vi "IdleState.vi"(8 "error in (no error)":errorcluster, 9 "Cluster in":T2, 10 "Enum in":T1, 11 "Actual Start [i]":i64) -> (0 "error out":errorcluster, 2 "Cluster out":T2, 3 "Enum":T1)   [LabVIEW 2018]
uses:
  Type_Def/Type_Def Actuator Controls.ctl
  Type_Def/Type_Def ControlState.ctl
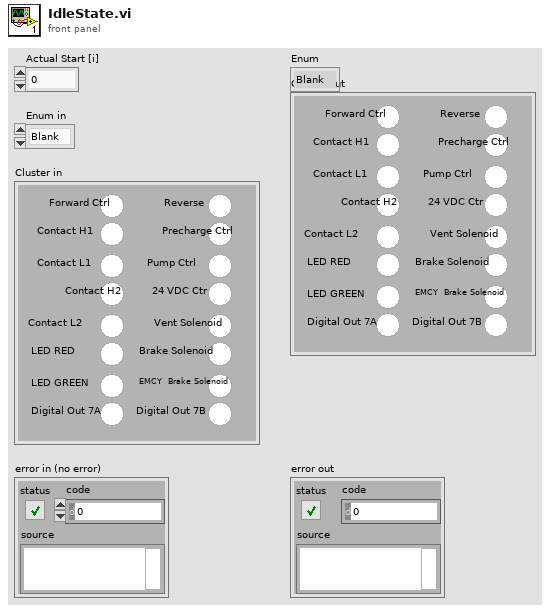
[diagram p1: front panel]
types:
  T1 = typedef "Type_Def ControlState.ctl" = enum16{"Blank", "Systems Check", "Idle", "Ready", "Pushing", "CrawlingPrecharge", "Braking", "Fault", "Boot Up", "Unpowered", "Crawling", "Shutdown", "Service Push", "Service Wait", "Vent", "Precharge", "Cooldown"}
  T2 = typedef "Type_Def Actuator Controls.ctl" = cluster{"Reverse ":bool, "Precharge Ctrl":bool, "Pump Ctrl":bool, "24 VDC Ctr":bool, "Vent Solenoid":bool, "Brake Solenoid":bool, "EMCY  Brake Solenoid":bool, "Digital Out 7B ":bool, "Forward Ctrl":bool, "Contact H1":bool, "Contact L1":bool, "Contact H2":bool, "Contact L2 ":bool, "LED RED":bool, "LED GREEN":bool, " Digital Out 7A":bool}
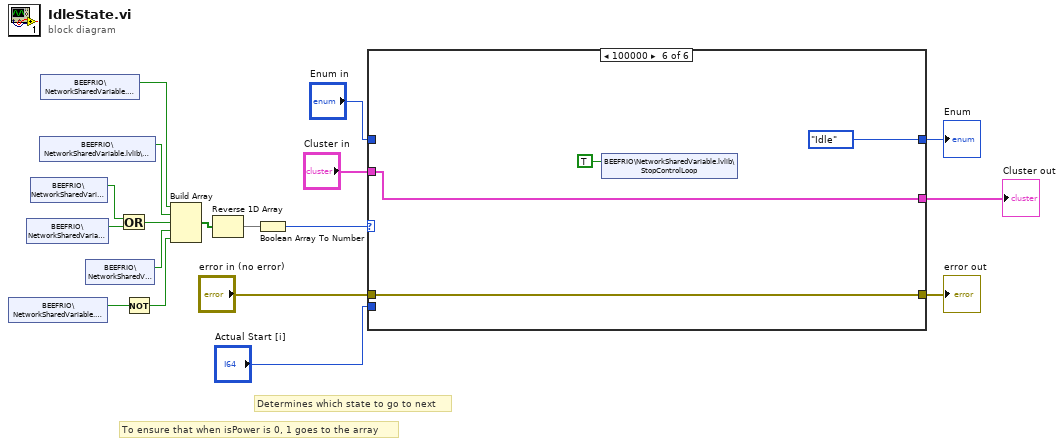
[diagram p0: block diagram]
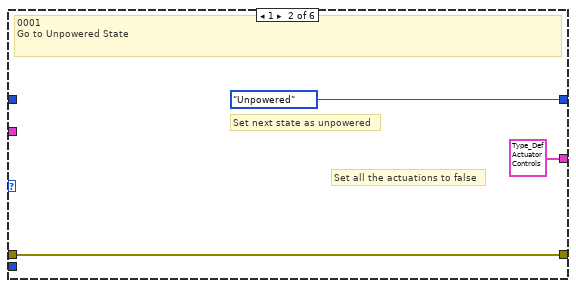
[diagram p3: hidden frame]
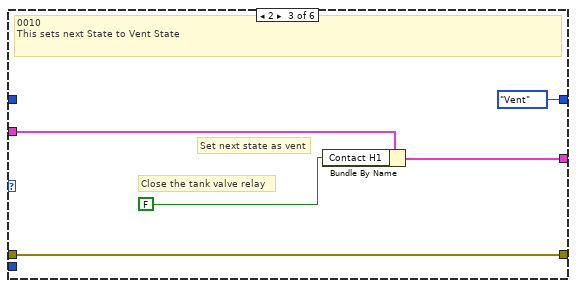
[diagram p4: hidden frame]
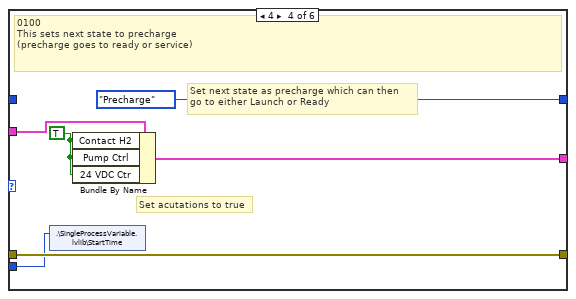
[diagram p5: hidden frame]
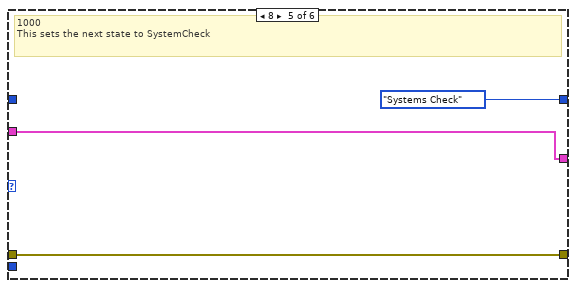
[diagram p6: hidden frame]
diagram:
  # "To ensure that when isPower is 0, 1 goes to the array"
  # "Determines which state to go to next"
  n1 = shared-variable "BEEFRIO\\NetworkSharedVariable.lvlib\\IsPowered"() -> (w11:bool)  [unwired: 1 in, 1 out]
  n2 = shared-variable "BEEFRIO\\NetworkSharedVariable.lvlib\\Service"() -> (w13:bool)  [unwired: 1 in, 1 out]
  n3 = shared-variable "BEEFRIO\\NetworkSharedVariable.lvlib\\Ready"() -> (w14:bool)  [unwired: 1 in, 1 out]
  n4 = shared-variable "BEEFRIO\\NetworkSharedVariable.lvlib\\SystemCheck"() -> (w2:bool)  [unwired: 1 in, 1 out]
  n5 = shared-variable "BEEFRIO\\NetworkSharedVariable.lvlib\\Shutdown"() -> (w1:bool)  [unwired: 1 in, 1 out]
  n6 = shared-variable "BEEFRIO\\NetworkSharedVariable.lvlib\\Vent"() -> (w7:bool)  [unwired: 1 in, 1 out]
  n7 = Or(x=w14, y=w13) -> (x .or. y?=w15:bool)
  n8 = Not(x=w11) -> (.not. x?=w12:bool)
  n9 = Build Array(w1, w2, w15, w7, w12) -> (w8:bool[])
  n10 = Reverse 1D Array(array=w8) -> (reversed array=w9:bool[])
  n11 = Boolean Array To Number(Boolean array=w9) -> (number=w10:u32)
  n12 = case shown="100000" w10 {
    tunnel: "Enum in" -> [w21 _ _ _ _ _]
    tunnel: [w21 Type_Def_ControlState."Unpowered" Type_Def_ControlState."Vent" Type_Def_ControlState."Precharge" Type_Def_ControlState."Systems Check" Type_Def_ControlState."Idle" ("Enum in")] -> w4
    tunnel: "Cluster in" -> [w20 _ w26 w34 w37 w42]
    tunnel: [w20 T2 {"Reverse "=FALSE, "Precharge Ctrl"=FALSE, "Pump Ctrl"=FALSE, "24 VDC Ctr"=FALSE, "Vent Solenoid"=FALSE, "Brake Solenoid"=FALSE, "EMCY  Brake Solenoid"=FALSE, "Digital Out 7B "=FALSE, "Forward Ctrl"=FALSE, "Contact H1"=FALSE, "Contact L1"=FALSE, "Contact H2"=FALSE, "Contact L2 "=FALSE, "LED RED"=FALSE, "LED GREEN"=FALSE, " Digital Out 7A"=FALSE} w27 w32 w37 w42] -> w6
    tunnel: [w19 w22 w25 w31 w36 w40] -> w16
    tunnel: "error in (no error)" -> [w19 w22 w25 w31 w36 w40]
    tunnel: "Actual Start [i]" -> [_ _ _ w30 _ _]
    frame 0, Default {
      # "Does nothing and stays in Idle mode"
    }
    frame 1 {
      # "Set next state as unpowered"
      # "Set all the actuations to false"
      # "0001\nGo to Unpowered State"
    }
    frame 2 {
      # "Set next state as vent"
      # "Close the tank valve relay"
      # "0010\nThis sets next State to Vent State"
      n13 = Bundle By Name(cluster=w26, "Contact H1"=FALSE) -> (w27:T2)
    }
    frame 4 {
      w33 = TRUE
      # "Set next state as precharge which can then \ngo to either Launch or Ready"
      # "Set acutations to true"
      # "0100\nThis sets next state to precharge \n(precharge goes to ready or service)"
      n14 = shared-variable ".\\SingleProcessVariable.lvlib\\StartTime"(w30) -> ()  [unwired: 1 in, 1 out]
      n15 = Bundle By Name(cluster=w34, "Contact H2"=w33, "Pump Ctrl"=w33, "24 VDC Ctr"=w33) -> (w32:T2)
    }
    frame 8 {
      # "1000\nThis sets the next state to SystemCheck"
    }
    frame 32 {
      n16 = shared-variable "BEEFRIO\\NetworkSharedVariable.lvlib\\StopControlLoop"(TRUE ("StopControlLoop")) -> ()  [unwired: 1 in, 1 out]
    }
  }
  "error out" <- w16
  "Cluster out" <- w6
  "Enum" <- w4
